vi "tic_tac_toe.vi"   [LabVIEW 2016]
uses:
  <vilib>/NXT/Block Support/NXT_ButtonSelector.ctl
  <vilib>/NXT/Block Support/NXT_InputPort.ctl
  <vilib>/NXT/Subs/ColorSensorColors.ctl
  <vilib>/NXT/Block Support/NXT_OutputPort.ctl
  <vilib>/NXT/NXTIO Xnodes/NXTIONodeSubVIs/NXTStopMotors.vi
  <vilib>/NXT/NXTIO Xnodes/NXTIONodeSubVIs/LEGOResetMotors.vi
  <vilib>/NXT/NXTIO Xnodes/NXTIONodeSubVIs/NXTMoveMotors.vi
  <vilib>/NXT/NXTIO Xnodes/NXTIONodeSubVIs/LEGOMotorStatus.vi
  <vilib>/NXT/Subs/LVHSConnector.ctl
  <vilib>/NXT/NXTIO Xnodes/AddressXNode/NXTIOAddress.xnode
  <vilib>/NXT/NXTIO Xnodes/NXTIOXNode/NXTIO.xnode
  <vilib>/NXT/LegoClasses/BrickReference/BrickReference.lvclass
types:
  T1 = enum16{"move3_2", "move3_3", "move3_4", "move3_5"}
  T2 = enum16{"Bereit", "Move 1", "Reference_pos", "Wait", "row1_check", "row2_check", "row3_check", "return", "move2", "move3", "move4", "move5", "end"}
  T3 = typedef "ColorSensorColors.ctl" = enum16{"No Color", "Black", "Blue", "Green", "Yellow", "Red", "White", "Brown"}
  T4 = typedef "NXT_OutputPort.ctl" = u8
  T5 = cluster{"Output Port":T4, "Output Port 2":T4, "Output Port 3":T4}
  T6 = typedef "NXT_ButtonSelector.ctl" = u16
  T7 = typedef "NXT_InputPort.ctl" = u32
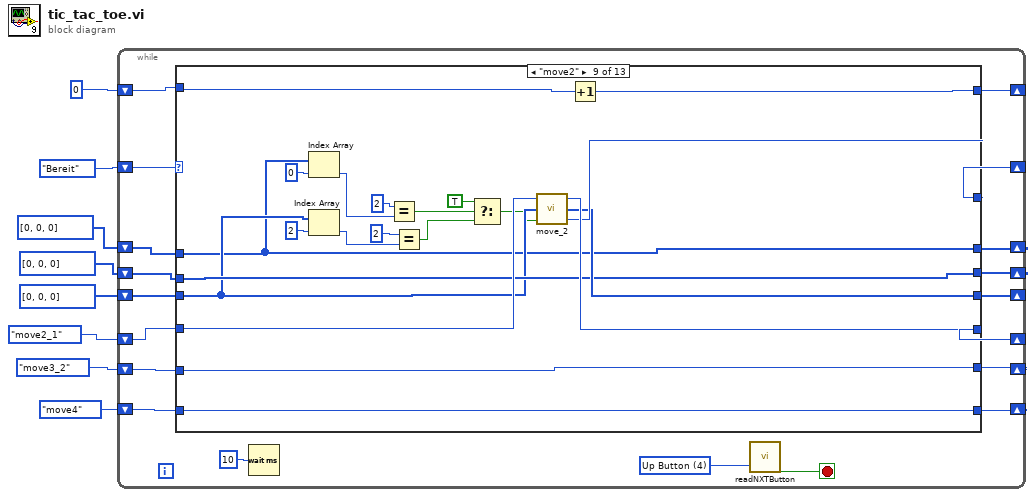
[diagram p0: block diagram]
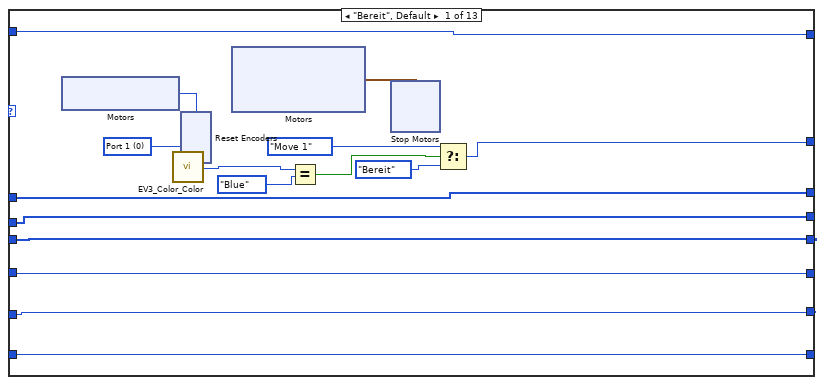
[diagram p2: hidden frame]
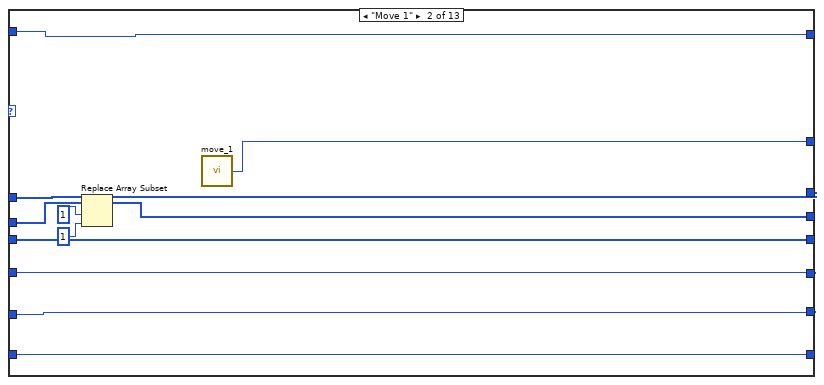
[diagram p3: hidden frame]
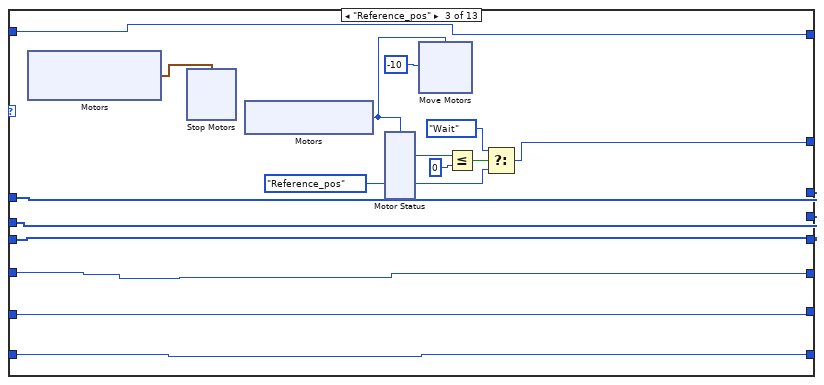
[diagram p4: hidden frame]
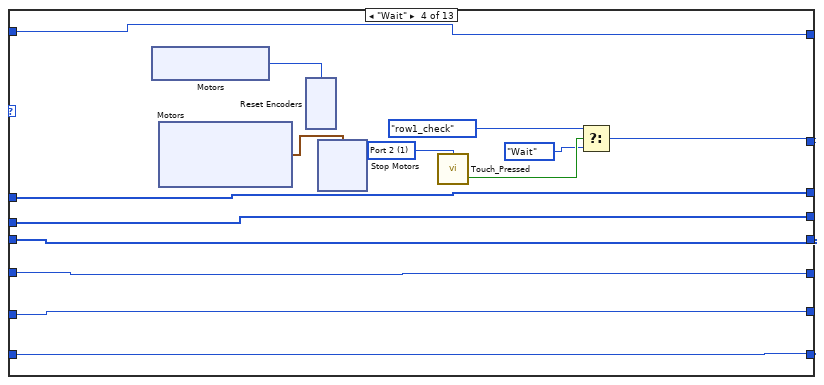
[diagram p5: hidden frame]
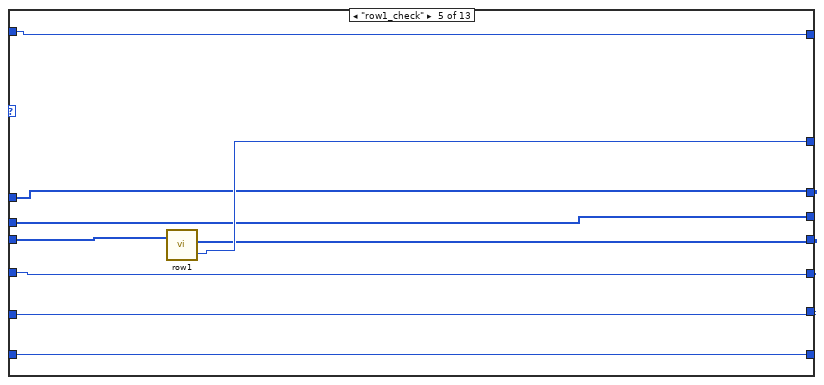
[diagram p6: hidden frame]
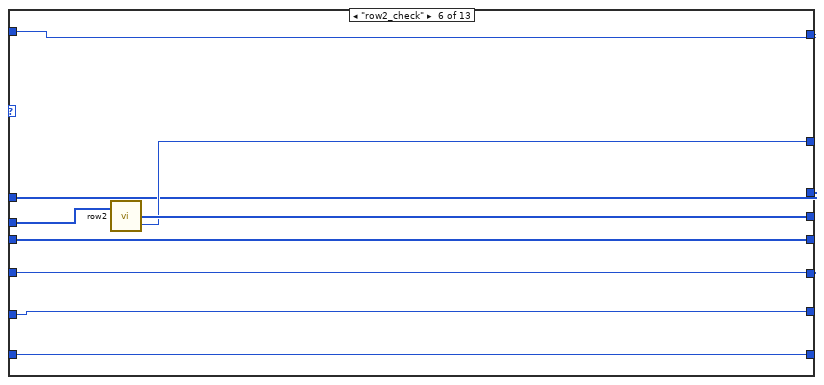
[diagram p7: hidden frame]
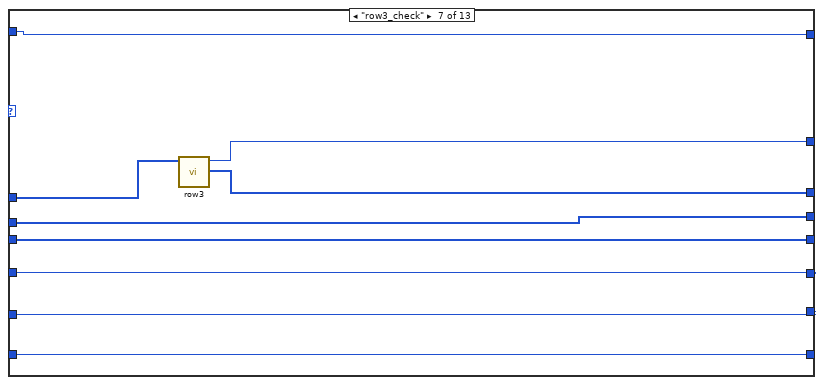
[diagram p8: hidden frame]
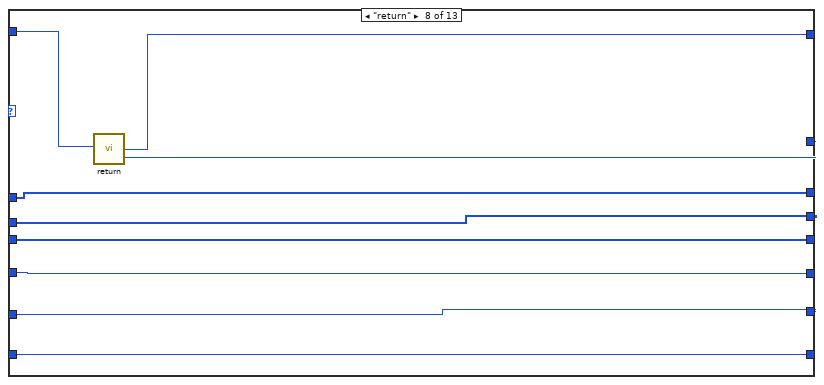
[diagram p9: hidden frame]
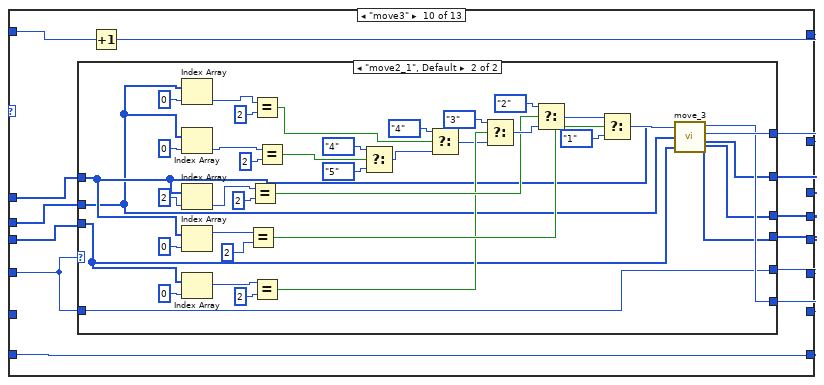
[diagram p10: hidden frame]
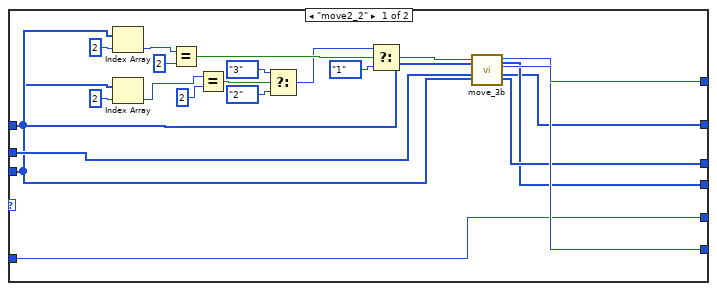
[diagram p11: hidden frame]
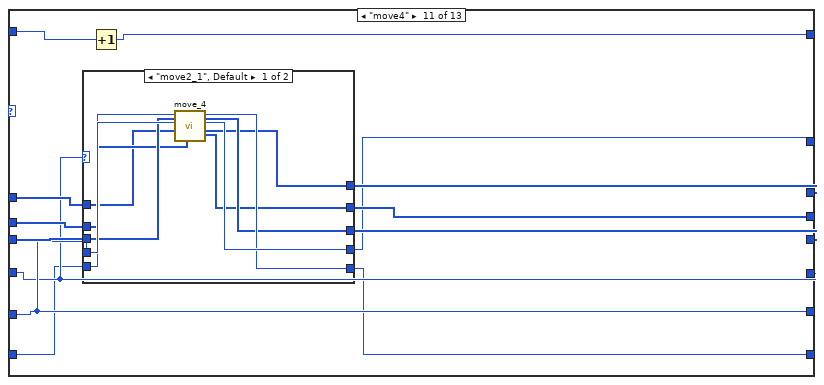
[diagram p12: hidden frame]
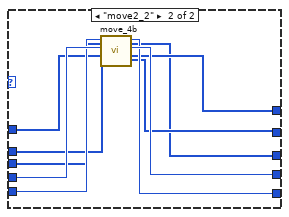
[diagram p13: hidden frame]
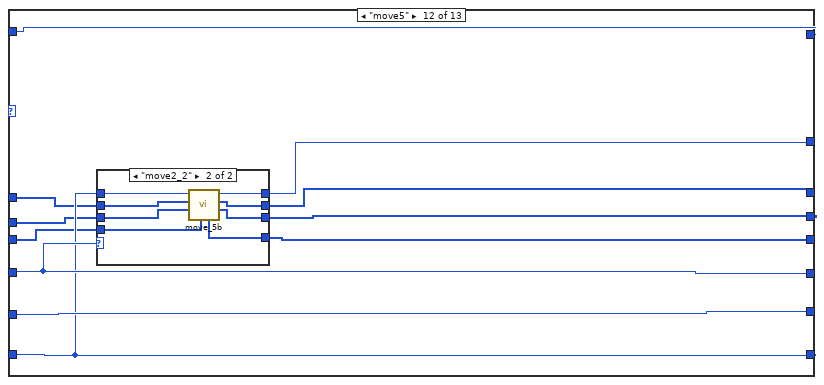
[diagram p14: hidden frame]
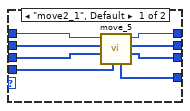
[diagram p15: hidden frame]
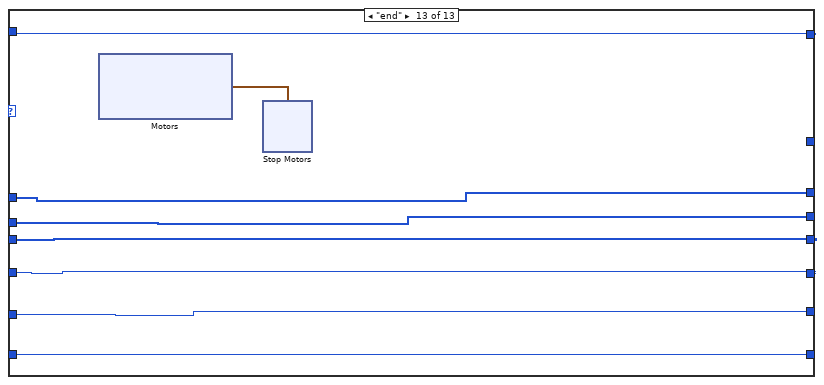
[diagram p16: hidden frame]
diagram:
  n1 = while {
    shift-right: [w23] -> _
    shift-left: T2."Bereit" -> [w24]
    shift-right: [w18] -> _
    shift-left: enum16{"move2_1", "move2_2"}."move2_1" -> [w17]
    shift-right: [w20] -> _
    shift-left: T1."move3_2" -> [w19]
    shift-right: [w22] -> _
    shift-left: enum16{"move4", "move4_1", "move4_2"}."move4" -> [w21]
    shift-right: [w13] -> _
    shift-left: i32[] [0, 0, 0] -> [w15]
    shift-right: [w16] -> _
    shift-left: i32[] [0, 0, 0] -> [w12]
    shift-right: [w14] -> _
    shift-left: i32[] [0, 0, 0] -> [w11]
    shift-right: [w9] -> _
    shift-left: 0 ("y") -> [w10]
    stop <- w25 stop-if-true
    w26 = T6 4 items=["Enter button"=3, "Left button"=2, "Right button"=1, "Up Button"=4, "Down Button"=5] ("Button (Enter button)")
    n2 = case shown="\"move2\"" w24 {
      tunnel: [w37 w65 w69 w112 w136 w144 w155 w164 w181 w186 w262 w300 _] -> w23
      tunnel: [w36 w62 w71 w108 w137 w141 w152 w161 w182 w187 w263 w301 w324] -> w22
      tunnel: w21 -> [w36 w62 w71 w108 w137 w141 w152 w161 w182 w187 w261 w301 w324]
      tunnel: [w35 w63 w72 w109 w135 w142 w153 w162 w184 w190 w265 w302 w325] -> w20
      tunnel: w19 -> [w35 w63 w72 w109 w135 w142 w153 w162 w184 _ w265 w302 w325]
      tunnel: [w34 w64 w73 w110 w134 w143 w154 w163 w183 w189 w264 w303 w326] -> w18
      tunnel: w17 -> [w34 w64 w73 w110 w134 w143 w154 w163 w185 w188 w264 w303 w326]
      tunnel: [w33 w58 w70 w111 w132 w145 w149 w159 w179 w193 w269 w296 w322] -> w13
      tunnel: w15 -> [w33 w61 w70 w111 w132 w146 w149 w159 w179 w194 w268 w299 w322]
      tunnel: [w32 w57 w68 w107 w131 w139 w150 w160 w174 w192 w267 w295 w323] -> w16
      tunnel: w12 -> [w32 w57 w68 w107 w131 w139 w151 w160 w174 w198 w266 w294 w323]
      tunnel: [w31 w56 w67 w106 w133 w140 w148 w158 w180 w191 w270 w298 w321] -> w14
      tunnel: w11 -> [w31 w56 w67 w106 w130 w140 w148 w158 w177 w197 w271 w297 w321]
      tunnel: w10 -> [w30 w55 w66 w105 w129 w138 w147 w157 w166 w196 w273 w304 w328]
      tunnel: [w30 w55 w66 w105 w129 w138 w147 w156 w165 w195 w272 w304 w328] -> w9
      frame "Bereit", Default {
        w41 = T7 0 items=["Port 1", "Port 2", "Port 3", "Port 4"] ("Port (Port 3)")
        n3 = xnode "Motors"() -> ("Motor"=w29:T4)
        n4 = call <vilib>:"EV3_Color_Color.vi"("Port (Port 1)"=w41) -> ("Detected Color"=w40:T3)  [unwired: 2 in, 1 out]
        n5 = xnode "Reset Encoders"("Motors"=w29) -> ()  [unwired: 1 in, 1 out]
        n6 = xnode "Motors"() -> ("Motor"=w28:cluster{"Port":T4, "Port":T4, "Port":T4})
        n7 = Equal?(x=w40, y=ColorSensorColors."Blue") -> (x = y?=w42:bool)
        n8 = xnode "Stop Motors"("Motors"=w28) -> ()  [unwired: 1 in, 1 out]
        n9 = Select(t=T2."Move 1", s=w42, f=T2."Bereit") -> (s? t:f=w37:T2)
      }
      frame "Move 1" {
        n10 = Replace Array Subset(array=w61, new element=1 ("disabled index (col)"), index=1 ("index (row)")) -> (w58:i32[])
        n11 = call "move_1.vi"() -> ("Enum"=w65:T2)  [unwired: 2 in]
      }
      frame "Reference_pos" {
        n12 = xnode "Motors"() -> ("Motor"=w81:cluster{"Port":T4, "Port":T4})
        n13 = xnode "Stop Motors"("Motors"=w81) -> ()  [unwired: 1 in, 1 out]
        n14 = xnode "Motors"() -> ("Motor"=w79:T4)
        n15 = xnode "Motor Status"("Motors"=w79) -> ("Position 1"=w78:i32)  [unwired: 1 in, 2 out]
        n16 = xnode "Move Motors"("Power/Speed 1"=i8 -10, "Motors"=w79) -> ()  [unwired: 1 in, 1 out]
        n17 = Less Or Equal?(x=w78, y=0) -> (x <= y?=w76:bool)
        n18 = Select(t=T2."Wait", s=w76, f=T2."Reference_pos") -> (s? t:f=w69:T2)
      }
      frame "Wait" {
        w117 = T7 1 items=["Port 1", "Port 2", "Port 3", "Port 4"] ("Port (Port 1)")
        n19 = xnode "Motors"() -> ("Motor"=w104:T4)
        n20 = xnode "Motors"() -> ("Motor"=w113:cluster{"Port":T4, "Port":T4, "Port":T4})
        n21 = xnode "Reset Encoders"("Motors"=w104) -> ()  [unwired: 1 in, 1 out]
        n22 = xnode "Stop Motors"("Motors"=w113) -> ()  [unwired: 1 in, 1 out]
        n23 = call <vilib>:"Touch_Pressed.vi"("Port (Port 1)"=w117) -> ("Yes / No"=w116:bool)  [unwired: 2 in, 1 out]
        n24 = Select(t=T2."row1_check", s=w116, f=T2."Wait") -> (s? t:f=w112:T2)
      }
      frame "row1_check" {
        n25 = call "row1.vi"("Array in"=w130) -> ("Array out"=w133:i32[], "Enum"=w136:T2)
      }
      frame "row2_check" {
        n26 = call "row2.vi"("Array in"=w146) -> ("Array out"=w145:i32[], "Enum"=w144:T2)
      }
      frame "row3_check" {
        n27 = call "row3.vi"("Array in"=w151) -> ("Array out"=w150:i32[], "Enum"=w155:T2)  [unwired: 9 in]
      }
      frame "return" {
        n28 = call "return.vi"("y in"=w157) -> ("y out"=w156:i32, "Enum"=w164:T2)
      }
      frame "move2" {
        n29 = Index Array(array=w174, index=0) -> (element=w172:i32)
        n30 = Index Array(array=w177, index=2) -> (element=w176:i32)
        n31 = Equal?(x=2, y=w172) -> (x = y?=w170:bool)
        n32 = Equal?(x=2, y=w176) -> (x = y?=w169:bool)
        n33 = Select(t=TRUE, s=w170, f=w169) -> (s? t:f=w168:bool)
        n34 = call "move_2.vi"("t"=w168, "Array in"=w177, "Enum 3"=w185) -> ("Enum"=w181:T2, "Array out"=w180:i32[], "Enum 2"=w183:enum16{"move2_1", "move2_2"})
        n35 = Increment(x=w166) -> (x+1=w165:i32)
      }
      frame "move3" {
        n36 = case shown="\"move2_1\", Default" w188 {
          tunnel: [w214 w251] -> w186
          tunnel: [w213 w250] -> w190
          tunnel: w198 -> [w207 w225]
          tunnel: w197 -> [w203 w223]
          tunnel: w194 -> [w205 w222]
          tunnel: [w206 w227] -> w193
          tunnel: [w199 w226] -> w192
          tunnel: [w204 w224] -> w191
          tunnel: [w202 w221] -> w189
          tunnel: w188 -> [w202 w221]
          frame "move2_2" {
            n37 = Index Array(array=w207, index=2) -> (element=w211:i32)
            n38 = Index Array(array=w203, index=2) -> (element=w209:i32)
            n39 = Equal?(x=w211, y=2 ("element")) -> (x = y?=w220:bool)
            n40 = Equal?(x=w209, y=2 ("element")) -> (x = y?=w217:bool)
            n41 = Select(t=enum16{"1", "2", "3"}."3", s=w217, f=enum16{"1", "2", "3"}."2") -> (s? t:f=w215:enum16{"1", "2", "3"})
            n42 = Select(t=w215, s=w220, f=enum16{"1", "2", "3"}."1") -> (s? t:f=w208:enum16{"1", "2", "3"})
            n43 = call "move_3b.vi"("Array in"=w203, "Array 3"=w205, "Array 5"=w207, "Enum in"=w208) -> ("Array 6"=w199:i32[], "Enum 3"=w214:T2, "Enum out"=w213:T1, "Array 4"=w206:i32[], "Array out"=w204:i32[])  [unwired: 3 in]
          }
          frame "move2_1", Default {
            n44 = Index Array(array=w222, index=0) -> (element=w237:i32)
            n45 = Index Array(array=w222, index=0) -> (element=w233:i32)
            n46 = Index Array(array=w225, index=2) -> (element=w246:i32)
            n47 = Index Array(array=w225, index=0) -> (element=w248:i32)
            n48 = Index Array(array=w223, index=0) -> (element=w241:i32)
            n49 = Equal?(x=w248, y=2 ("element")) -> (x = y?=w260:bool)
            n50 = Equal?(x=w246, y=2 ("element")) -> (x = y?=w244:bool)
            n51 = Equal?(x=w237, y=2 ("element")) -> (x = y?=w238:bool)
            n52 = Equal?(x=w241, y=2) -> (x = y?=w240:bool)
            n53 = Equal?(x=w233, y=2 ("element")) -> (x = y?=w231:bool)
            n54 = Select(t=enum16{"1", "2", "3", "4", "5"}."4", s=w231, f=enum16{"1", "2", "3", "4", "5"}."5") -> (s? t:f=w229:enum16{"1", "2", "3", "4", "5"})
            n55 = Select(t=enum16{"1", "2", "3", "4", "5"}."4", s=w238, f=w229) -> (s? t:f=w230:enum16{"1", "2", "3", "4", "5"})
            n56 = Select(t=enum16{"1", "2", "3", "4", "5"}."3", s=w240, f=w230) -> (s? t:f=w254:enum16{"1", "2", "3", "4", "5"})
            n57 = Select(t=enum16{"1", "2", "3", "4", "5"}."2", s=w244, f=w254) -> (s? t:f=w256:enum16{"1", "2", "3", "4", "5"})
            n58 = Select(t=w256, s=w260, f=enum16{"1", "2", "3", "4", "5"}."1") -> (s? t:f=w252:enum16{"1", "2", "3", "4", "5"})
            n59 = call "move_3.vi"("Enum 3"=w252, "Array 3"=w225, "Array 6"=w222, "Array in"=w223) -> ("Array out"=w224:i32[], "Enum"=w250:T1, "Enum 2"=w251:T2, "Array 5"=w227:i32[], "Array 4"=w226:i32[])  [unwired: 2 in]
          }
        }
        n60 = Increment(x=w196) -> (x+1=w195:i32)
      }
      frame "move4" {
        n61 = case shown="\"move2_1\", Default" w264 {
          tunnel: w265 -> [w283 w293]
          tunnel: [w282 w292] -> w262
          tunnel: [w281 w291] -> w263
          tunnel: w261 -> [w280 w290]
          tunnel: w271 -> [w279 w284]
          tunnel: [w278 w285] -> w270
          tunnel: [w277 w289] -> w269
          tunnel: w268 -> [w276 w288]
          tunnel: [w275 w287] -> w267
          tunnel: w266 -> [w274 w286]
          frame "move2_1", Default {
            n62 = call "move_4.vi"("Array 3"=w276, "Array 6"=w279, "Array in"=w274, "Enum 4"=w283, "Enum in"=w280) -> ("Array out"=w275:i32[], "Enum 3"=w282:T2, "Enum out"=w281:enum16{"move4", "move4_1", "move4_2"}, "Array 4"=w277:i32[], "Array 5"=w278:i32[])  [unwired: 2 in]
          }
          frame "move2_2" {
            n63 = call "move_4b.vi"("Array 5"=w288, "Array in"=w284, "Array 3"=w286, "Enum 4"=w293, "Enum in"=w290) -> ("Array 4"=w287:i32[], "Enum 3"=w292:T2, "Enum out"=w291:enum16{"move4", "move4_1", "move4_2"}, "Array 6"=w289:i32[], "Array out"=w285:i32[])  [unwired: 2 in]
          }
        }
        n64 = Increment(x=w273) -> (x+1=w272:i32)
      }
      frame "move5" {
        n65 = case shown="\"move2_2\"" w303 {
          tunnel: w301 -> [w305 w320]
          tunnel: [w306 w319] -> w300
          tunnel: w299 -> [w312 w318]
          tunnel: [w311 w313] -> w298
          tunnel: w297 -> [w310 w314]
          tunnel: [w309 w317] -> w296
          tunnel: [w308 w316] -> w295
          tunnel: w294 -> [w307 w315]
          frame "move2_1", Default {
            n66 = call "move_5.vi"("Array 4"=w310, "Array 6"=w312, "Array in"=w307, "Enum in"=w305) -> ("Array 3"=w309:i32[], "Array out"=w308:i32[], "Enum out"=w306:T2, "Array 5"=w311:i32[])  [unwired: 4 in]
          }
          frame "move2_2" {
            n67 = call "move_5b.vi"("Array in"=w314, "Array 6"=w318, "Array 3"=w315, "Enum in"=w320) -> ("Array 5"=w317:i32[], "Array 4"=w316:i32[], "Enum out"=w319:T2, "Array out"=w313:i32[])  [unwired: 4 in]
          }
        }
      }
      frame "end" {
        n68 = xnode "Motors"() -> ("Motor"=w327:cluster{"Port":T4, "Port":T4, "Port":T4})
        n69 = xnode "Stop Motors"("Motors"=w327) -> ()  [unwired: 1 in, 1 out]
      }
    }
    n70 = Wait (ms)(milliseconds to wait=u32 10 ("Zu wartende ms")) -> ()  [unwired: 1 out]
    n71 = call <vilib>:"readNXTButton.vi"("Button (Enter button)"=w26) -> ("Yes/No"=w25:bool)  [unwired: 2 in, 1 out]
  }
